vi "Untitled 1.vi"() -> ()   [LabVIEW 2013]
uses:
  <vilib>/Utility/file.llb/Read From Spreadsheet File (DBL).vi
  <userlib>/caLab/Private/CaLabEvent_PV.vi
  <userlib>/caLab/Private/Put_DBL-1D_PV.vi
  <userlib>/caLab/Private/Put_I32_PV.vi
panel:
  out "XY Graph 3":cluster{"ID1:REF:X":dbl[], "all rows":dbl[]}[](graph)
  out "XY Graph 2":cluster{"ID1:REF:X":dbl[], "all rows":dbl[]}[](graph)
  out "tag2":string
  out "tag1":string
  out "XY Graph":cluster{"ID1:REF:X":dbl[], "all rows":dbl[]}[](graph)
  in  "file path (dialog if empty)":path
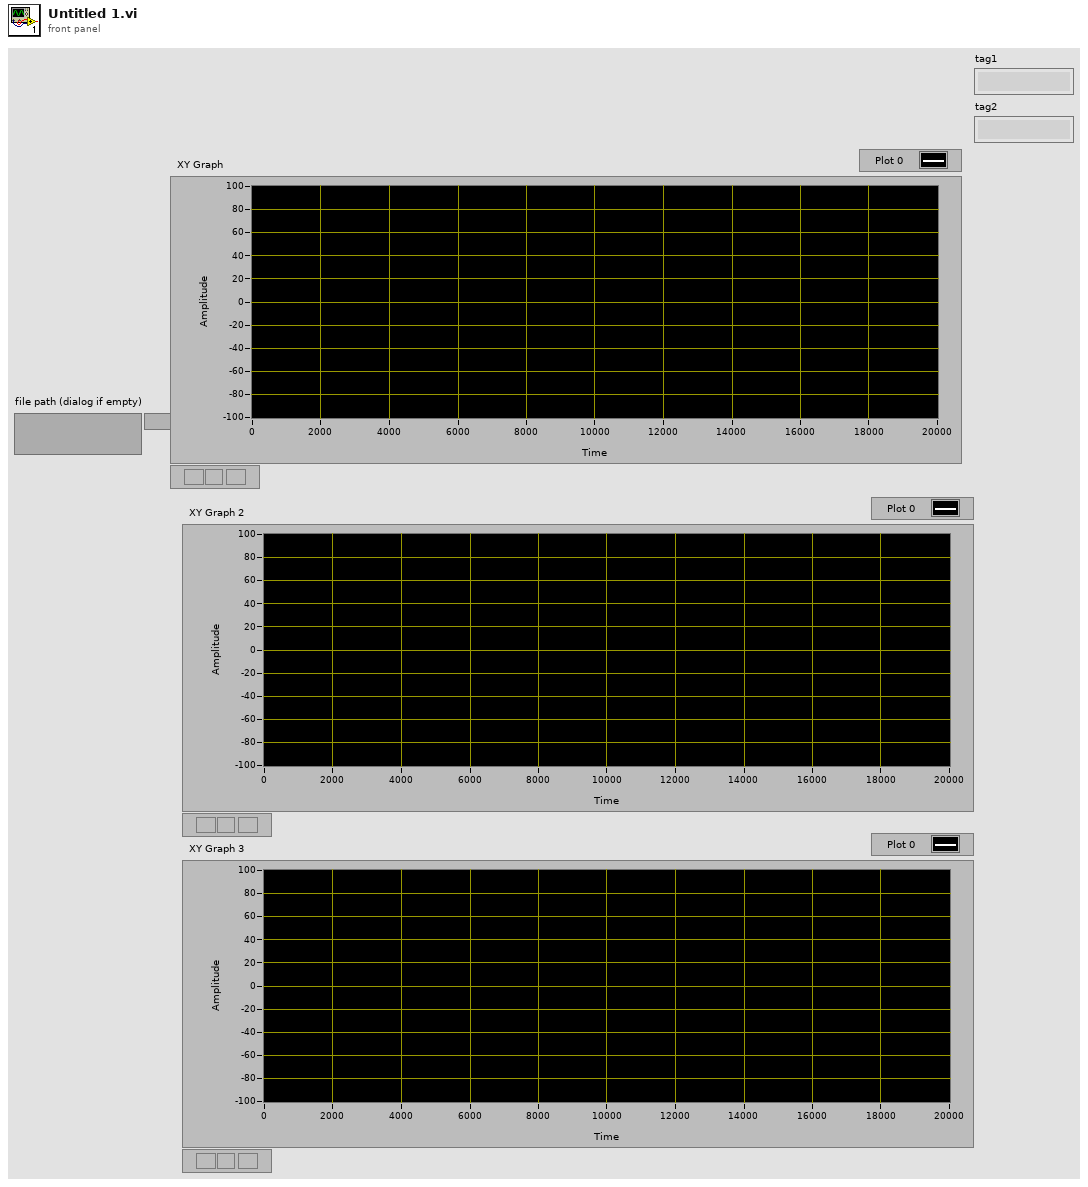
[diagram p1: front panel]
types:
  T1 = cluster{"tag1":string, "tag2":string, "x":dbl[], "y":dbl[], "ID1:X":dbl[], "ID1:Y":dbl[], "ID1:REF:X":dbl[], "ID1:REF:Y":dbl[], "ID2:X":dbl[], "ID2:Y":dbl[], "ID2:REF:X":dbl[], "ID2:REF:Y":dbl[], "ID3:X":dbl[], "ID3:Y":dbl[], "ID3:REF:X":dbl[], "ID3:REF:Y":dbl[], "ID1:TAG1":string, "ID1:TAG2":string, "ID2:TAG1":string, "ID2:TAG2":string, "ID3:TAG1":string, "ID3:TAG2":string, "ID1:NAME":string, "ID2:NAME":string, "ID3:NAME":string, "ID1:SCORE":string, "ID2:SCORE":string, "ID3:SCORE":string, "NO":string}
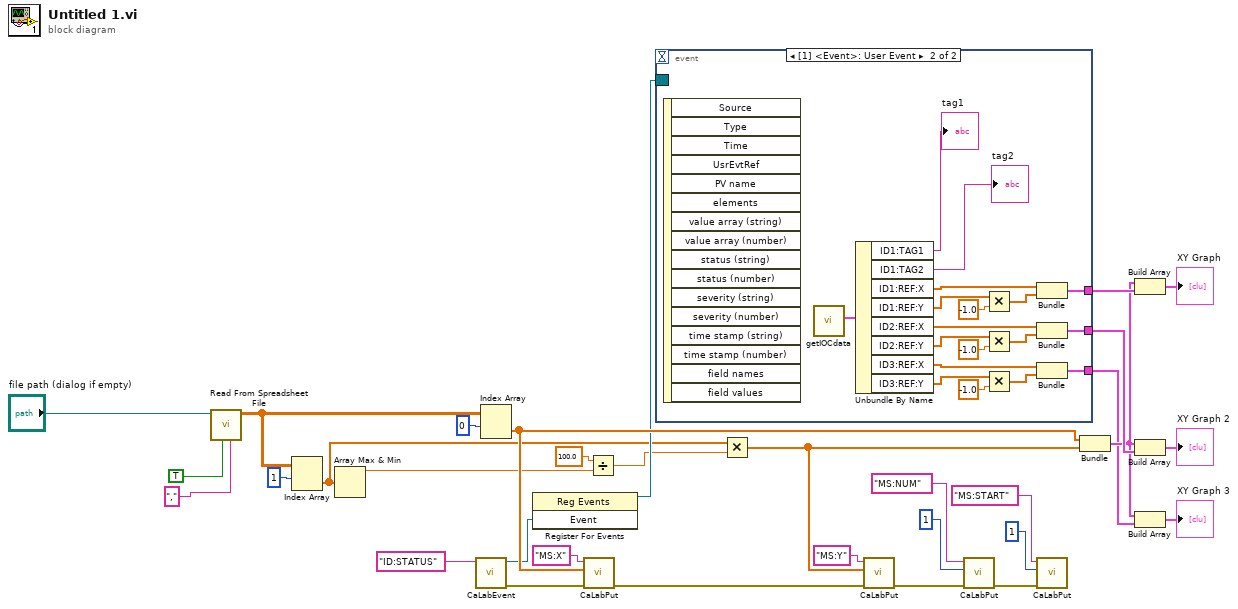
[diagram p0: block diagram]
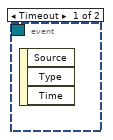
[diagram p2: hidden frame]
diagram:
  n1 = call-poly <vilib>:"Read From Spreadsheet File.vi"("delimiter (\\t)"="," ("delimiter (\\t)"), "transpose (no:F)"=TRUE, "file path (dialog if empty)"="file path (dialog if empty)") -> ("all rows"=w28:dbl[][])  [unwired: 4 in, 4 out]
  n2 = Index Array(array=w28, index (row)=1) -> (element=w7:dbl[])  [unwired: 1 in]
  n3 = Array Max & Min(array=w7) -> (max value=w9:dbl)  [unwired: 3 out]
  n4 = call-poly <userlib>:"CaLabEvent.vi"("PV Name"="ID:STATUS") -> ("error out"=w13:errorcluster, "Event"=w15:refnum<user-event>)  [unwired: 8 in, 1 out]
  n5 = Index Array(array=w28, index (row)=0) -> (element=w17:dbl[])  [unwired: 1 in]
  n6 = register-events(w15) -> (reference out=w14:refnum<event-registration>)  [unwired: 2 in, 1 out]
  n7 = call-poly <userlib>:"CaLabPut.vi"("Error in (no error)"=w13, "Values"=w17, "PV Names"="MS:X") -> ("Error out"=w25:errorcluster)  [unwired: 5 in, 3 out]
  n8 = Divide(x=100.0, y=w9) -> (x/y=w8:dbl)
  n9 = event shown="[1] <Event>: User Event" {
    selector: w14 -> [_ _]
    dyn-events: _ -> [_ _]
    timeout: _ -> [_ _]
    tunnel: [_ w46] -> w12
    tunnel: [_ w38] -> w5
    tunnel: [_ w33] -> w3
    event Timeout {
      n10 = event-data() -> ()  [unwired: 1 in, 3 out]
    }
    event User Event {
      n11 = event-data() -> ()  [unwired: 1 in, 16 out]
      n12 = call "getIOCdata.vi"() -> ("输出簇"=w50:T1)  [unwired: 11 in]
      n13 = Unbundle By Name(w50) -> ("ID1:TAG1"=→"tag1":string, "ID1:TAG2"=→"tag2":string, "ID1:REF:X"=w47:dbl[], "ID1:REF:Y"=w45:dbl[], "ID2:REF:X"=w42:dbl[], "ID2:REF:Y"=w41:dbl[], "ID3:REF:X"=w37:dbl[], "ID3:REF:Y"=w36:dbl[])
      n14 = Multiply(x=w45, y=-1.0) -> (x*y=w43:dbl[])
      n15 = Multiply(x=w41, y=-1.0) -> (x*y=w39:dbl[])
      n16 = Multiply(x=w36, y=-1.0) -> (x*y=w35:dbl[])
      n17 = Bundle("ID1:REF:X"=w47, w43) -> (w46:cluster{"ID1:REF:X":dbl[], dbl[]})  [unwired: 1 in]
      n18 = Bundle("ID2:REF:X"=w42, w39) -> (w38:cluster{"ID2:REF:X":dbl[], dbl[]})  [unwired: 1 in]
      n19 = Bundle("ID3:REF:X"=w37, w35) -> (w33:cluster{"ID3:REF:X":dbl[], dbl[]})  [unwired: 1 in]
    }
  }
  n20 = Multiply(x=w7, y=w8) -> (x*y=w6:dbl[])
  n21 = call-poly <userlib>:"CaLabPut.vi"("Error in (no error)"=w25, "Values"=w6, "PV Names"="MS:Y") -> ("Error out"=w23:errorcluster)  [unwired: 5 in, 3 out]
  n22 = call-poly <userlib>:"CaLabPut.vi"("Error in (no error)"=w23, "Value"=1, "PV Name"="MS:NUM") -> ("Error out"=w22:errorcluster)  [unwired: 5 in, 3 out]
  n23 = call-poly <userlib>:"CaLabPut.vi"("Error in (no error)"=w22, "Value"=1, "PV Name"="MS:START") -> ()  [unwired: 5 in, 4 out]
  n24 = Bundle("all rows"=w17, w6) -> (w4:cluster{"all rows":dbl[], dbl[]})  [unwired: 1 in]
  n25 = Build Array(w4, w12) -> (→"XY Graph":cluster{"ID1:REF:X":dbl[], dbl[]}[])
  n26 = Build Array(w4, w5) -> (→"XY Graph 2":cluster{"ID2:REF:X":dbl[], dbl[]}[])
  n27 = Build Array(w4, w3) -> (→"XY Graph 3":cluster{"ID3:REF:X":dbl[], dbl[]}[])
